vi "record_tsv_CCP_tmp.vi"(1 "use_nfs_disk_also":bool=TRUE, 2 "use_date_folder":bool=TRUE, 3 "logging_on":bool=TRUE, 5 "file_name":string="record", 6 "error in":errorcluster, 7 "folder_name":string="subsystem", 8 "format_array":string[](array[string]), 9 "value_array":dbl[](array[numeric])=[0.0], 10 "format":string, 11 "time":timestamp) -> (0 "status":bool, 4 "error out":errorcluster)   [LabVIEW 2019]
uses:
  <vilib>/Utility/file.llb/Write Delimited Spreadsheet (string).vi
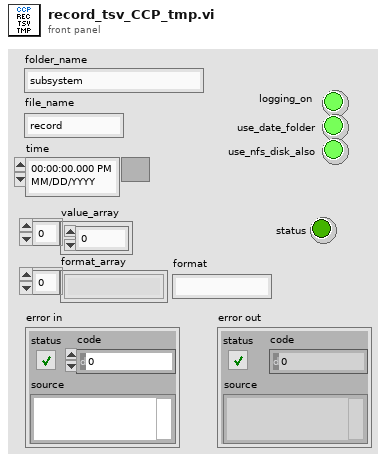
[diagram p1: front panel]
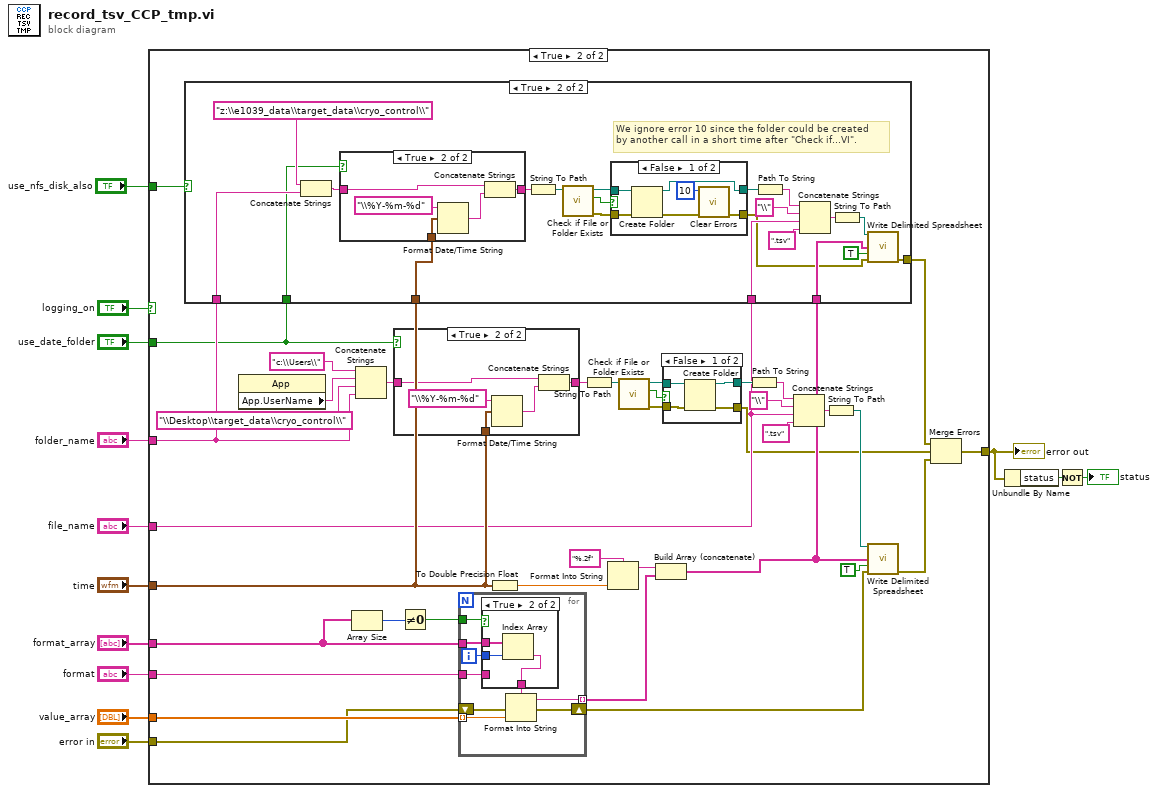
[diagram p0: block diagram]
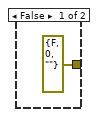
[diagram p3: hidden frame]
diagram:
  n1 = case shown="True" "logging_on" {
    tunnel: "file_name" -> [_ w24]
    tunnel: "folder_name" -> [_ w26]
    tunnel: "value_array" -> [_ w35]
    tunnel: [w14 w20] -> w4
    tunnel: "format_array" -> [_ w31]
    tunnel: "use_date_folder" -> [_ w22]
    tunnel: "time" -> [_ w25]
    tunnel: "error in" -> [w14 w28]
    tunnel: "use_nfs_disk_also" -> [_ w21]
    tunnel: "format" -> [_ w15]
    frame False {
    }
    frame True {
      n2 = property class="App"() -> ("App.UserName"=w48:string)  [unwired: 2 in, 2 out]
      n3 = Array Size(array=w31) -> (size(s)=w30:i32)
      n4 = Concatenate Strings("c:\\Users\\", w48, "\\Desktop\\target_data\\cryo_control\\", w26) -> (w33:string)
      n5 = case shown="True" w22 {
        tunnel: w33 -> [w88 w93]
        tunnel: [w88 w92] -> w32
        tunnel: w25 -> [_ w91]
        frame False {
        }
        frame True {
          n6 = Format Date/Time String(time format string (%c)="\\%Y-%m-%d", seconds (now)=w91) -> (date/time string=w89:string)  [unwired: 1 in]
          n7 = Concatenate Strings(w93, w89) -> (w92:string)
        }
      }
      n8 = Not Equal To 0?(x=w30) -> (x != 0?=w29:bool)
      n9 = for {
        tunnel: [w102] -> w34 mode=indexing
        tunnel: w35 -> [w101] mode=indexing
        tunnel: w31 -> [w98]
        tunnel: w29 -> [w100]
        shift-right: [w96] -> w27
        shift-left: w28 -> [w97]
        tunnel: w15 -> [w94]
        i -> [w95]
        n10 = case shown="True" w100 {
          tunnel: [w103 w106] -> w99
          tunnel: w98 -> [_ w105]
          tunnel: w95 -> [_ w104]
          tunnel: w94 -> [w103 _]
          frame False {
          }
          frame True {
            n11 = Index Array(array=w105, index=w104) -> (element=w106:string)
          }
        }
        n12 = Format Into String(format string=w99, error in=w97, w101) -> (resulting string=w102:string, error out=w96:errorcluster)  [unwired: 1 in]
      }
      n13 = To Double Precision Float(number=w25) -> (double precision float=w37:dbl)
      n14 = String To Path(string=w32) -> (path=w43:path)
      n15 = Format Into String(format string="%.2f", w37) -> (resulting string=w51:string)  [unwired: 2 in, 1 out]
      n16 = call <vilib>:"Check if File or Folder Exists.vi"("path"=w43) -> ("error out"=w19:errorcluster, "file or folder exists?"=w42:bool, "dup path"=w40:path)  [unwired: 8 in]
      n17 = Build Array (concatenate)(w51, w34) -> (w23:string[])
      n18 = case shown="True" w21 {
        tunnel: w26 -> [_ w62]
        tunnel: w25 -> [_ w61]
        tunnel: w24 -> [_ w60]
        tunnel: w23 -> [_ w57]
        tunnel: w22 -> [_ w56]
        tunnel: [errorcluster {"status"=FALSE, "code"=0, "source"=""} ("error out") w53] -> w16
        frame False {
        }
        frame True {
          # "We ignore error 10 since the folder could be created\nby another call in a short time after \"Check if...VI\"."
          n19 = Concatenate Strings("z:\\e1039_data\\target_data\\cryo_control\\", w62) -> (w64:string)
          n20 = case shown="True" w56 {
            tunnel: w64 -> [w74 w79]
            tunnel: [w74 w78] -> w63
            tunnel: w61 -> [_ w77]
            frame False {
            }
            frame True {
              n21 = Format Date/Time String(time format string (%c)="\\%Y-%m-%d", seconds (now)=w77) -> (date/time string=w75:string)  [unwired: 1 in]
              n22 = Concatenate Strings(w79, w75) -> (w78:string)
            }
          }
          n23 = String To Path(string=w63) -> (path=w69:path)
          n24 = call <vilib>:"Check if File or Folder Exists.vi"("path"=w69) -> ("error out"=w55:errorcluster, "file or folder exists?"=w68:bool, "dup path"=w66:path)  [unwired: 8 in]
          n25 = case shown="False" w68 {
            tunnel: w66 -> [w85 w87]
            tunnel: [w84 w87] -> w67
            tunnel: w55 -> [w83 w86]
            tunnel: [w81 w86] -> w54
            frame False {
              n26 = Create Folder(path (use dialog)=w85, error in=w83) -> (created path=w84:path, error out=w82:errorcluster)  [unwired: 1 in, 1 out]
              n27 = call <vilib>:"Clear Errors.vi"("error in (no error)"=w82, "specific error code to clear (0: all)"=10) -> ("error out"=w81:errorcluster)  [unwired: 4 in, 1 out]
            }
            frame True {
            }
          }
          n28 = Path To String(path=w67) -> (string=w65:string)
          n29 = Concatenate Strings(w65, "\\", w60, ".tsv" ("string")) -> (w70:string)
          n30 = String To Path(string=w70) -> (path=w59:path)
          n31 = call-poly <vilib>:"Write Delimited Spreadsheet.vi"("file path (dialog if empty)"=w59, "1D data"=w57, "append to file? (new file:F)"=TRUE, "error in (no error)"=w54) -> ("error out"=w53:errorcluster)  [unwired: 10 in, 1 out]
        }
      }
      n32 = case shown="False" w42 {
        tunnel: w40 -> [w110 w112]
        tunnel: [w109 w112] -> w41
        tunnel: w19 -> [w108 w111]
        tunnel: [w107 w111] -> w18
        frame False {
          n33 = Create Folder(path (use dialog)=w110, error in=w108) -> (created path=w109:path, error out=w107:errorcluster)  [unwired: 1 in, 1 out]
        }
        frame True {
        }
      }
      n34 = Path To String(path=w41) -> (string=w39:string)
      n35 = Concatenate Strings(w39, "\\", w24, ".tsv" ("string")) -> (w44:string)
      n36 = String To Path(string=w44) -> (path=w38:path)
      n37 = call-poly <vilib>:"Write Delimited Spreadsheet.vi"("file path (dialog if empty)"=w38, "1D data"=w23, "append to file? (new file:F)"=TRUE, "error in (no error)"=w27) -> ("error out"=w17:errorcluster)  [unwired: 10 in, 1 out]
      n38 = Merge Errors(w16, w18, w17) -> (w20:errorcluster)
    }
  }
  "error out" <- w4
  n39 = Unbundle By Name(w4) -> ("status"=w3:bool)
  n40 = Not(x=w3) -> (.not. x?=→"status":bool)
